vi "io_attr_query.vi"(5 "Read Long data for ViString (F)":bool, 7 "Attribute":T1={"Identifier"="", "Descriptive name"="", "Data Type"=enum."Integer 32", "Command"="", "Access"=2, "Range Table"="", "Read Callback"="", "Write Callback"="", "Range Callback"="", "Check Callback"="", "Rngtable Callback"="", "Coerce Callback"="", "Supported Models"="", "Instrument Options"="", "Repeated Capabilities"="", "Check Status Callback"="", "Index"=0, "Flag: OPC Wait"=FALSE, "Flag: Dont check status"=FALSE, "Flag: Cache Only"=FALSE} {"Access" items=["Read Only", "Write Only", "Read/Write"]}, 8 "error in":errorcluster, 10 "write buffer":string, 11 "VISA resource name":refnum<visa-resource-name>) -> (0 "error out":errorcluster, 2 "read buffer":string, 3 "VISA resource name out":refnum<visa-resource-name>)   [LabVIEW 2014, in "rszvl_rsidr_core.lvlib"]
uses:
  rszvl_rsidr_core.lvlib
  type_Attribute.ctl
  type_Attribute_Data_Type.ctl
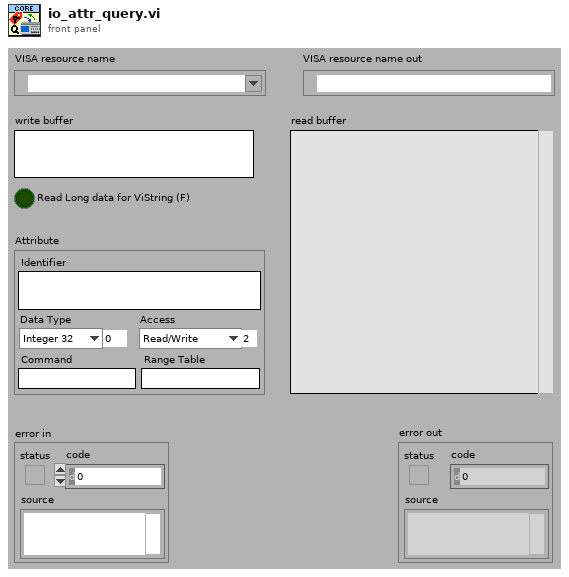
[diagram p1: front panel]
types:
  T1 = typedef "rszvl_rsidr_core.lvlib/type_Attribute.ctl" = cluster{"Identifier":string, "Descriptive name":string, "Data Type":T2, "Command":string, "Access":u16, "Range Table":string, "Read Callback":string, "Write Callback":string, "Range Callback":string, "Check Callback":string, "Rngtable Callback":string, "Coerce Callback":string, "Supported Models":string, "Instrument Options":string, "Repeated Capabilities":string, "Check Status Callback":string, "Index":i32, "Flag: OPC Wait":bool, "Flag: Dont check status":bool, "Flag: Cache Only":bool}
  T2 = typedef "rszvl_rsidr_core.lvlib/type_Attribute_Data_Type.ctl" = enum16{"Integer 32", "Double", "String", "Boolean", "None", "Integer 64"}
  T3 = enum16{"Initialize", "Check", "Get Numeric Value", "Get Default Value"}
  T4 = typedef "rszvl_rsidr_core.lvlib/type_Session_Data.ctl" = cluster{"Instr type":string, "Instr type for err. msg.":string, "Installed Options":string[], "OPC Timeout":i32, "Query Instrument Status":bool, "Check Range":bool, "Check Options":bool, "Add LF to Write":bool, "Simulate":bool, "Logging":bool, "Logging params":variant, "Interface Type":enum16{"Unknown", "GPIB", "VXI", "GPIB_VXI", "ASRL", "PXI", "TCPIP", "USB", "SOCKET"}, "Fast Sweep":i32, "AdditionalFlags":i32, "WaitBeforeWrite":i32, "WaitBeforeRead":i32, "BinDataChunkSize":i64}
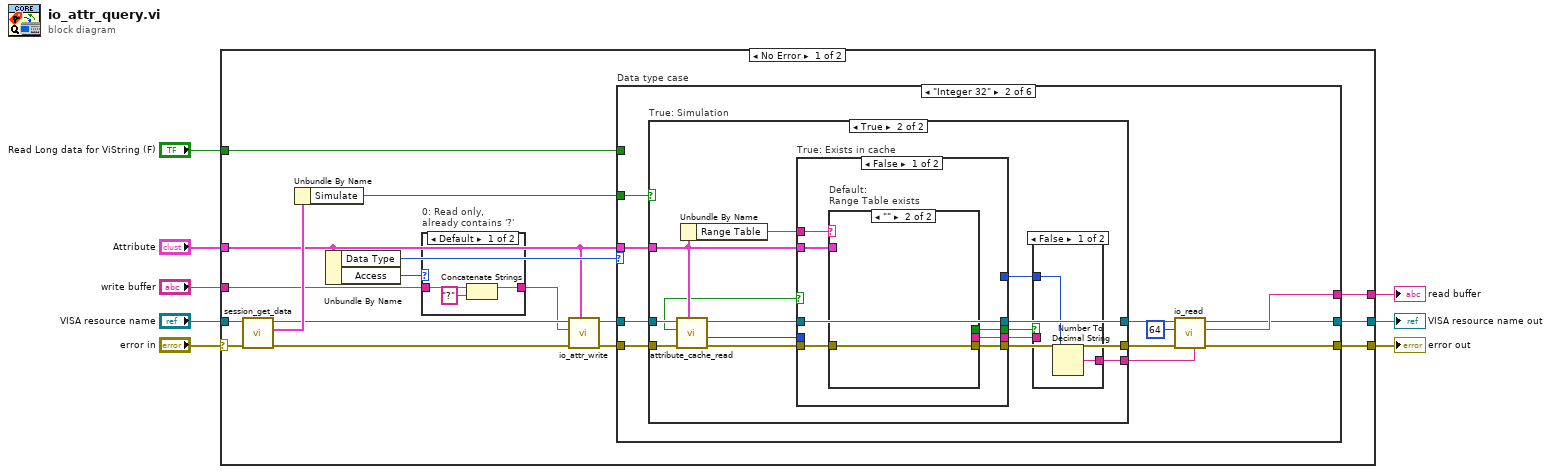
[diagram p0: block diagram]
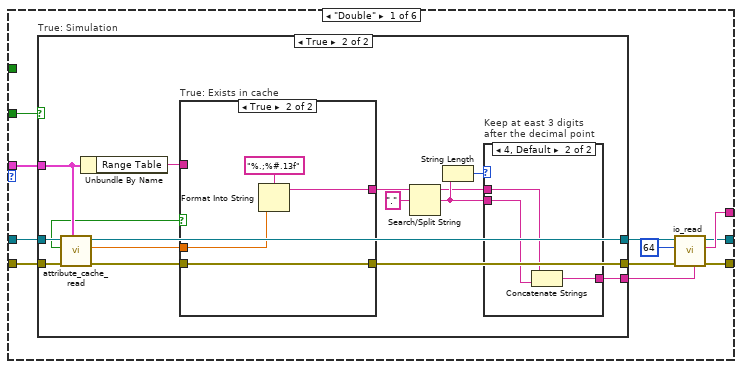
[diagram p3: hidden frame]
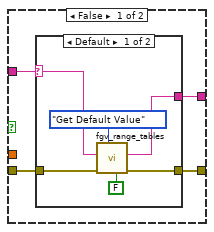
[diagram p5: hidden frame]
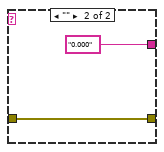
[diagram p6: hidden frame]
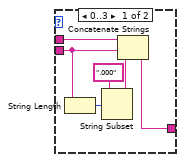
[diagram p7: hidden frame]
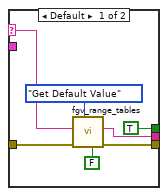
[diagram p9: hidden frame]
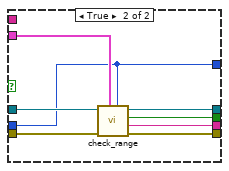
[diagram p10: hidden frame]
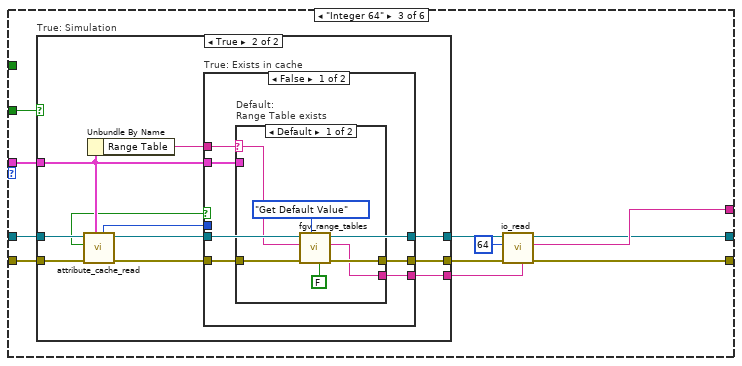
[diagram p12: hidden frame]
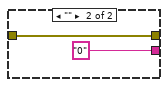
[diagram p14: hidden frame]
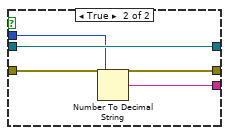
[diagram p15: hidden frame]
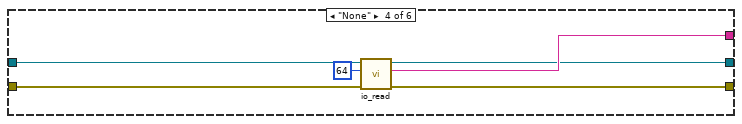
[diagram p16: hidden frame]
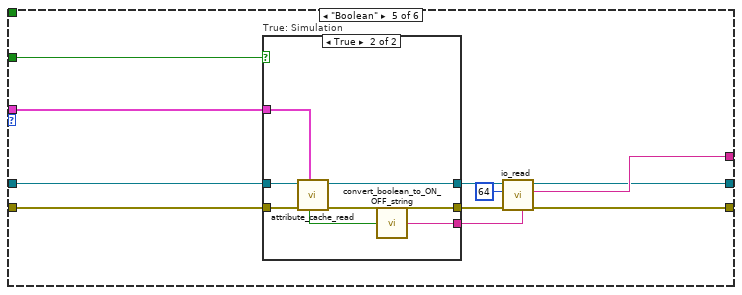
[diagram p17: hidden frame]
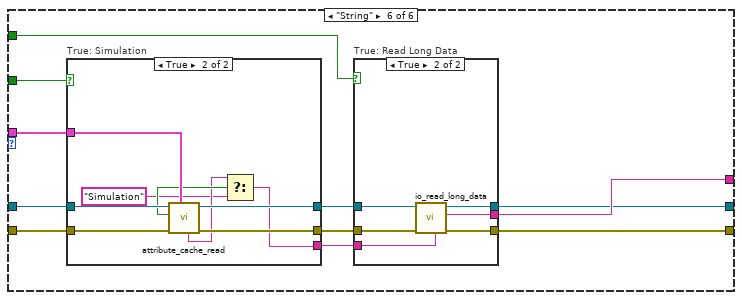
[diagram p19: hidden frame]
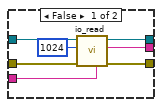
[diagram p20: hidden frame]
diagram:
  n1 = case shown="No Error" "error in" {
    selector: "error in" -> [w18 w240]
    tunnel: "VISA resource name" -> [w17 w239]
    tunnel: [w22 w240] -> w5
    tunnel: [w21 w239] -> w4
    tunnel: [w24 _] -> w8
    tunnel: "write buffer" -> [w12 _]
    tunnel: "Attribute" -> [w9 _]
    tunnel: "Read Long data for ViString (F)" -> [w11 _]
    frame No Error {
      n2 = call "session_get_data.vi"("error in"=w18, "VISA resource name"=w17) -> ("error out"=w16:errorcluster, "Session User Data out"=w23:T4, "VISA resource name out"=w15:refnum<visa-resource-name>)  [unwired: 7 in]
      n3 = Unbundle By Name(w23) -> ("Simulate"=w19:bool)
      n4 = Unbundle By Name(w9) -> ("Data Type"=w20:T2, "Access"=w25:u16)
      n5 = case "0: Read only,\nalready contains '?'" shown="Default" w25 {
        tunnel: [w26 w29] -> w10
        tunnel: w12 -> [w27 w29]
        frame Default {
          n6 = Concatenate Strings(w27, "?" ("string")) -> (w26:string)
        }
        frame 0 {
        }
      }
      n7 = call "io_attr_write.vi"("Attribute"=w9, "error in"=w16, "write buffer"=w10, "VISA resource name"=w15) -> ("error out"=w14:errorcluster, "VISA resource name out"=w13:refnum<visa-resource-name>)  [unwired: 6 in]
      n8 = case "Data type case" shown="\"Integer 32\"" w20 {
        tunnel: [w40 w93 w146 w183 w194 w214] -> w24
        tunnel: w14 -> [w35 w84 w137 w179 w189 w210]
        tunnel: w13 -> [w34 w83 w136 w178 w188 w209]
        tunnel: [w39 w92 w145 w182 w193 w213] -> w22
        tunnel: [w38 w91 w144 w181 w192 w212] -> w21
        tunnel: w19 -> [w36 w85 w138 _ w190 w211]
        tunnel: w9 -> [w31 w86 w139 _ w185 w206]
        tunnel: w11 -> [_ _ _ _ _ w204]
        frame "Double" {
          n9 = case "True: Simulation" shown="True" w36 {
            tunnel: w35 -> [w42 w57]
            tunnel: w34 -> [w41 w56]
            tunnel: [w41 w55] -> w33
            tunnel: [w42 w47] -> w32
            tunnel: w31 -> [_ w46]
            tunnel: [_ w50] -> w30
            frame False {
            }
            frame True {
              n10 = call "attribute_cache_read.vi"("Attribute"=w46, "error in"=w57, "VISA resource name"=w56) -> ("error out"=w49:errorcluster, "Double out"=w48:dbl, "VISA resource name out"=w55:refnum<visa-resource-name>, "Exists in cache"=w43:bool)  [unwired: 1 in, 4 out]
              n11 = Unbundle By Name(w46) -> ("Range Table"=w45:string)
              n12 = case "True: Exists in cache" shown="True" w43 {
                tunnel: w49 -> [w59 w70]
                tunnel: w48 -> [_ w71]
                tunnel: [w58 w70] -> w47
                tunnel: [w60 w72] -> w44
                tunnel: w45 -> [w61 _]
                frame False {
                  n13 = case shown="Default" w61 {
                    selector: w61 -> [w63 _]
                    tunnel: [w65 "0.000"] -> w60
                    tunnel: w59 -> [w67 w68]
                    tunnel: [w66 w68] -> w58
                    frame Default {
                      n14 = call "fgv_range_tables.vi"("Range Checking"=FALSE, "Operation"=T3."Get Default Value", "error in"=w67, "Range Table ID in"=w63) -> ("error out"=w66:errorcluster, "Default value out"=w65:string)  [unwired: 4 in, 2 out]
                    }
                    frame "" {
                    }
                  }
                }
                frame True {
                  n15 = Format Into String(format string="%.;%#.13f", w71) -> (resulting string=w72:string)  [unwired: 2 in, 1 out]
                }
              }
              n16 = Search/Split String(string=w44, search string/char (-)=".") -> (substring before match=w52:string, match + rest of string=w53:string)  [unwired: 1 in, 1 out]
              n17 = String Length(string=w53) -> (length=w54:i32)
              n18 = case "Keep at east 3 digits\nafter the decimal point" shown="4, Default" w54 {
                tunnel: w53 -> [w75 w80]
                tunnel: w52 -> [w79 w82]
                tunnel: [w78 w81] -> w50
                frame 0..3 {
                  n19 = String Length(string=w75) -> (length=w76:i32)
                  n20 = String Subset(string=".000", offset (0)=w76) -> (substring=w77:string)  [unwired: 1 in]
                  n21 = Concatenate Strings(w79, w75, w77) -> (w78:string)
                }
                frame 4, Default {
                  n22 = Concatenate Strings(w82, w80) -> (w81:string)
                }
              }
            }
          }
          n23 = call "io_read.vi"("Simulation read buffer (\"Simulation\")"=w30, "error in"=w32, "byte count (2048)"=u32 64 ("Max read bytes count (1024)"), "VISA resource name"=w33) -> ("error out"=w39:errorcluster, "read buffer"=w40:string, "VISA resource name out"=w38:refnum<visa-resource-name>)  [unwired: 4 in, 1 out]
        }
        frame "Integer 32" {
          n24 = case "True: Simulation" shown="True" w85 {
            tunnel: w84 -> [w95 w109]
            tunnel: w83 -> [w94 w108]
            tunnel: [w94 w96] -> w88
            tunnel: [w95 w105] -> w89
            tunnel: w86 -> [_ w106]
            tunnel: [_ w102] -> w87
            frame False {
            }
            frame True {
              n25 = call "attribute_cache_read.vi"("Attribute"=w106, "error in"=w109, "VISA resource name"=w108) -> ("error out"=w100:errorcluster, "Integer 32 out"=w101:i32, "VISA resource name out"=w97:refnum<visa-resource-name>, "Exists in cache"=w99:bool)  [unwired: 1 in, 4 out]
              n26 = Unbundle By Name(w106) -> ("Range Table"=w107:string)
              n27 = case "True: Exists in cache" shown="False" w99 {
                tunnel: w107 -> [w116 _]
                tunnel: w106 -> [w115 w130]
                tunnel: [w114 w126] -> w105
                tunnel: [w113 w127] -> w104
                tunnel: [w111 w128] -> w103
                tunnel: w101 -> [_ w125]
                tunnel: w100 -> [w112 w132]
                tunnel: [_ w125] -> w98
                tunnel: w97 -> [w110 w131]
                tunnel: [w110 w129] -> w96
                frame False {
                  n28 = case "Default:\nRange Table exists" shown="\"\"" w116 {
                    selector: w116 -> [w120 _]
                    tunnel: [w121 w124] -> w114
                    tunnel: w115 -> [_ _]
                    tunnel: [w119 _] -> w113
                    tunnel: w112 -> [w122 w124]
                    tunnel: [TRUE _] -> w111
                    frame Default {
                      n29 = call "fgv_range_tables.vi"("Range Checking"=FALSE, "Operation"=T3."Get Default Value", "error in"=w122, "Range Table ID in"=w120) -> ("error out"=w121:errorcluster, "Default value out"=w119:string)  [unwired: 4 in, 2 out]
                    }
                    frame "" {
                    }
                  }
                }
                frame True {
                  n30 = call "check_range.vi"("Attribute Value"=w125, "Attribute"=w130, "error in"=w132, "VISA resource name"=w131) -> ("error out"=w126:errorcluster, "Enum output"=w127:string, "Enum?"=w128:bool, "VISA resource name out"=w129:refnum<visa-resource-name>)  [unwired: 4 in]
                }
              }
              n31 = case shown="False" w103 {
                tunnel: w98 -> [w133 _]
                tunnel: w104 -> [_ w135]
                tunnel: [w134 w135] -> w102
                frame False {
                  n32 = Number To Decimal String(number=w133) -> (decimal integer string=w134:string)  [unwired: 1 in]
                }
                frame True {
                }
              }
            }
          }
          n33 = call "io_read.vi"("Simulation read buffer (\"Simulation\")"=w87, "error in"=w89, "byte count (2048)"=u32 64 ("Max read bytes count (1024)"), "VISA resource name"=w88) -> ("error out"=w92:errorcluster, "read buffer"=w93:string, "VISA resource name out"=w91:refnum<visa-resource-name>)  [unwired: 4 in, 1 out]
        }
        frame "Integer 64" {
          n34 = case "True: Simulation" shown="True" w138 {
            tunnel: w137 -> [w148 w159]
            tunnel: w136 -> [w147 w158]
            tunnel: [w147 w151] -> w141
            tunnel: [w148 w155] -> w142
            tunnel: w139 -> [_ w156]
            tunnel: [_ w150] -> w140
            frame False {
            }
            frame True {
              n35 = call "attribute_cache_read.vi"("Attribute"=w156, "error in"=w159, "VISA resource name"=w158) -> ("error out"=w154:errorcluster, "VISA resource name out"=w152:refnum<visa-resource-name>, "Integer 64 out"=w149:i64, "Exists in cache"=w153:bool)  [unwired: 1 in, 4 out]
              n36 = Unbundle By Name(w156) -> ("Range Table"=w157:string)
              n37 = case "True: Exists in cache" shown="False" w153 {
                tunnel: w157 -> [w165 _]
                tunnel: w156 -> [w164 _]
                tunnel: [w163 w176] -> w155
                tunnel: [w162 w177] -> w150
                tunnel: w149 -> [_ w174]
                tunnel: w154 -> [w161 w176]
                tunnel: w152 -> [w160 w175]
                tunnel: [w160 w175] -> w151
                frame False {
                  n38 = case "Default:\nRange Table exists" shown="Default" w165 {
                    selector: w165 -> [w168 _]
                    tunnel: [w169 w173] -> w163
                    tunnel: w164 -> [_ _]
                    tunnel: [w167 "0"] -> w162
                    tunnel: w161 -> [w170 w173]
                    frame Default {
                      n39 = call "fgv_range_tables.vi"("Range Checking"=FALSE, "Operation"=T3."Get Default Value", "error in"=w170, "Range Table ID in"=w168) -> ("error out"=w169:errorcluster, "Default value out"=w167:string)  [unwired: 4 in, 2 out]
                    }
                    frame "" {
                    }
                  }
                }
                frame True {
                  n40 = Number To Decimal String(number=w174) -> (decimal integer string=w177:string)  [unwired: 1 in]
                }
              }
            }
          }
          n41 = call "io_read.vi"("Simulation read buffer (\"Simulation\")"=w140, "error in"=w142, "byte count (2048)"=u32 64 ("Max read bytes count (1024)"), "VISA resource name"=w141) -> ("error out"=w145:errorcluster, "read buffer"=w146:string, "VISA resource name out"=w144:refnum<visa-resource-name>)  [unwired: 4 in, 1 out]
        }
        frame "None" {
          n42 = call "io_read.vi"("error in"=w179, "byte count (2048)"=u32 64 ("Max read bytes count (1024)"), "VISA resource name"=w178) -> ("error out"=w182:errorcluster, "read buffer"=w183:string, "VISA resource name out"=w181:refnum<visa-resource-name>)  [unwired: 5 in, 1 out]
        }
        frame "Boolean" {
          n43 = case "True: Simulation" shown="True" w190 {
            tunnel: w189 -> [w196 w203]
            tunnel: w188 -> [w195 w202]
            tunnel: [w195 w201] -> w187
            tunnel: [w196 w199] -> w186
            tunnel: w185 -> [_ w200]
            tunnel: [_ w197] -> w184
            frame False {
            }
            frame True {
              n44 = call "attribute_cache_read.vi"("Attribute"=w200, "error in"=w203, "VISA resource name"=w202) -> ("error out"=w199:errorcluster, "VISA resource name out"=w201:refnum<visa-resource-name>, "Boolean out"=w198:bool)  [unwired: 1 in, 5 out]
              n45 = call "convert_boolean_to_ON_OFF_string.vi"("boolean value in"=w198) -> ("string value out"=w197:string)  [unwired: 4 in]
            }
          }
          n46 = call "io_read.vi"("Simulation read buffer (\"Simulation\")"=w184, "error in"=w186, "byte count (2048)"=u32 64 ("Max read bytes count (1024)"), "VISA resource name"=w187) -> ("error out"=w193:errorcluster, "read buffer"=w194:string, "VISA resource name out"=w192:refnum<visa-resource-name>)  [unwired: 4 in, 1 out]
        }
        frame "String" {
          n47 = case "True: Simulation" shown="True" w211 {
            tunnel: w210 -> [w229 w238]
            tunnel: w209 -> [w228 w237]
            tunnel: [w228 w236] -> w208
            tunnel: [w229 w234] -> w207
            tunnel: w206 -> [_ w235]
            tunnel: [_ w233] -> w205
            frame False {
            }
            frame True {
              n48 = call "attribute_cache_read.vi"("Attribute"=w235, "error in"=w238, "VISA resource name"=w237) -> ("error out"=w234:errorcluster, "VISA resource name out"=w236:refnum<visa-resource-name>, "String out"=w231:string, "Exists in cache"=w232:bool)  [unwired: 1 in, 4 out]
              n49 = Select(t=w231, s=w232, f="Simulation") -> (s? t:f=w233:string)
            }
          }
          n50 = case "True: Read Long Data" shown="True" w204 {
            tunnel: [w221 w223] -> w214
            tunnel: [w220 w225] -> w213
            tunnel: [w219 w224] -> w212
            tunnel: w208 -> [w218 w226]
            tunnel: w207 -> [w217 w227]
            tunnel: w205 -> [w215 w222]
            frame False {
              n51 = call "io_read.vi"("Simulation read buffer (\"Simulation\")"=w215, "error in"=w217, "byte count (2048)"=u32 1024 ("byte count (1024)"), "VISA resource name"=w218) -> ("error out"=w220:errorcluster, "read buffer"=w221:string, "VISA resource name out"=w219:refnum<visa-resource-name>)  [unwired: 4 in, 1 out]
            }
            frame True {
              n52 = call "io_read_long_data.vi"("Simulation read buffer (\"Simulation\")"=w222, "error in"=w227, "VISA resource name"=w226) -> ("error out"=w225:errorcluster, "read buffer"=w223:string, "VISA resource name out"=w224:refnum<visa-resource-name>)  [unwired: 5 in, 1 out]
            }
          }
        }
      }
    }
    frame Error {
    }
  }
  "VISA resource name out" <- w4
  "error out" <- w5
  "read buffer" <- w8
